vi "controlTargetPosition.vi"(7 "Set":bool, 8 "error in":errorcluster, 9 "Target Position in":dbl, 10 "axis in":u8, 11 "connection ID":i32) -> (0 "error out":errorcluster, 1 "Target Position out":dbl, 2 "axis out":u8, 3 "connection ID":i32)   [LabVIEW 2016]
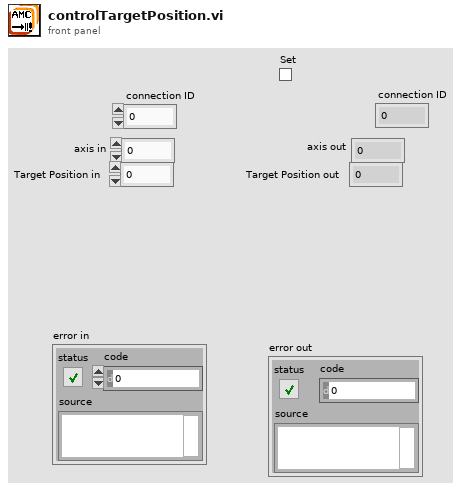
[diagram p1: front panel]
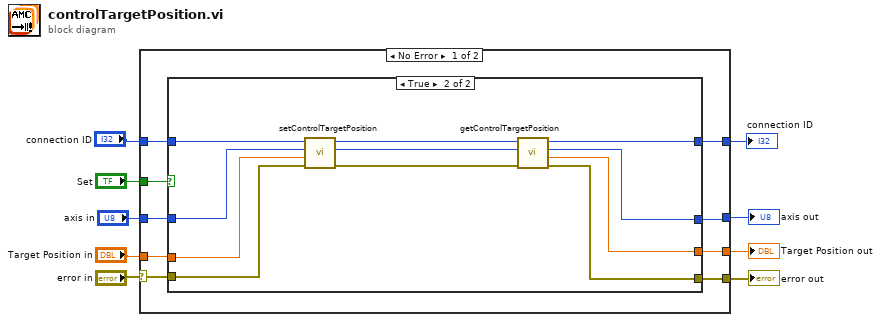
[diagram p0: block diagram]
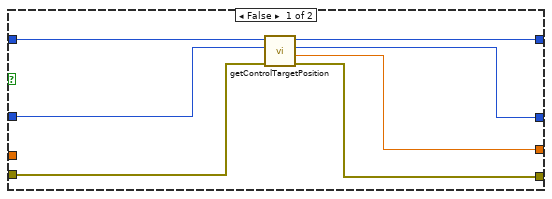
[diagram p2: hidden frame]
diagram:
  n1 = case shown="No Error" "error in" {
    selector: "error in" -> [w10 w40]
    tunnel: "axis in" -> [w15 w38]
    tunnel: [w11 w40] -> w8
    tunnel: [w13 w38] -> w7
    tunnel: "Target Position in" -> [w18 w39]
    tunnel: [w12 w39] -> w5
    tunnel: "Set" -> [w16 _]
    tunnel: [w14 w37] -> w3
    tunnel: "connection ID" -> [w17 w37]
    frame No Error {
      n2 = case shown="True" w16 {
        tunnel: [w21 w26] -> w14
        tunnel: w17 -> [w20 w36]
        tunnel: w15 -> [w19 w35]
        tunnel: [w22 w27] -> w13
        tunnel: [w24 w29] -> w11
        tunnel: [w23 w28] -> w12
        tunnel: w18 -> [_ w33]
        tunnel: w10 -> [w25 w34]
        frame False {
          n3 = call "getControlTargetPosition.vi"("error in"=w25, "axis"=w19, "connection ID"=w20) -> ("error out"=w24:errorcluster, "position"=w23:dbl, "axis_out"=w22:i32, "connection ID"=w21:i32)  [unwired: 5 in]
        }
        frame True {
          n4 = call "setControlTargetPosition.vi"("error in"=w34, "target"=w33, "axis"=w35, "connection ID"=w36) -> ("error out"=w30:errorcluster, "axis_out"=w31:i32, "connection ID"=w32:i32)  [unwired: 5 in]
          n5 = call "getControlTargetPosition.vi"("error in"=w30, "axis"=w31, "connection ID"=w32) -> ("error out"=w29:errorcluster, "position"=w28:dbl, "axis_out"=w27:i32, "connection ID"=w26:i32)  [unwired: 5 in]
        }
      }
    }
    frame Error {
    }
  }
  "error out" <- w8
  "axis out" <- w7
  "Target Position out" <- w5
  "connection ID" <- w3
